vi "Create trap overlay.vi"(0 "Current trap cluster":T1, 1 "Image in":T2, 2 "ROI size":dbl=24.0, 3 "Switch X/Y":bool, 4 "Path":T1[](array[typedef])) -> (5 "Image Out":T2)   [LabVIEW 8.6]
uses:
  <vilib>/vision/Image Controls.llb/IMAQ Image.ctl
  Trap cluster.ctl
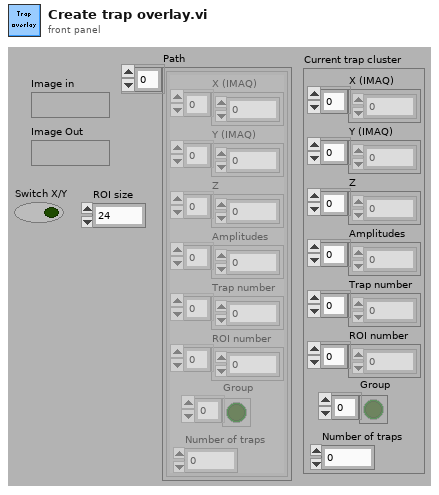
[diagram p1: front panel]
types:
  T1 = typedef "Trap cluster.ctl" = cluster{"X (IMAQ)":dbl[], "Y (IMAQ)":dbl[], "Z":dbl[], "Amplitudes":dbl[], "Trap number":i32[], "ROI number":i32[], "Number of traps":i32, "Group":bool[]}
  T2 = typedef "IMAQ Image.ctl" = refnum<image>
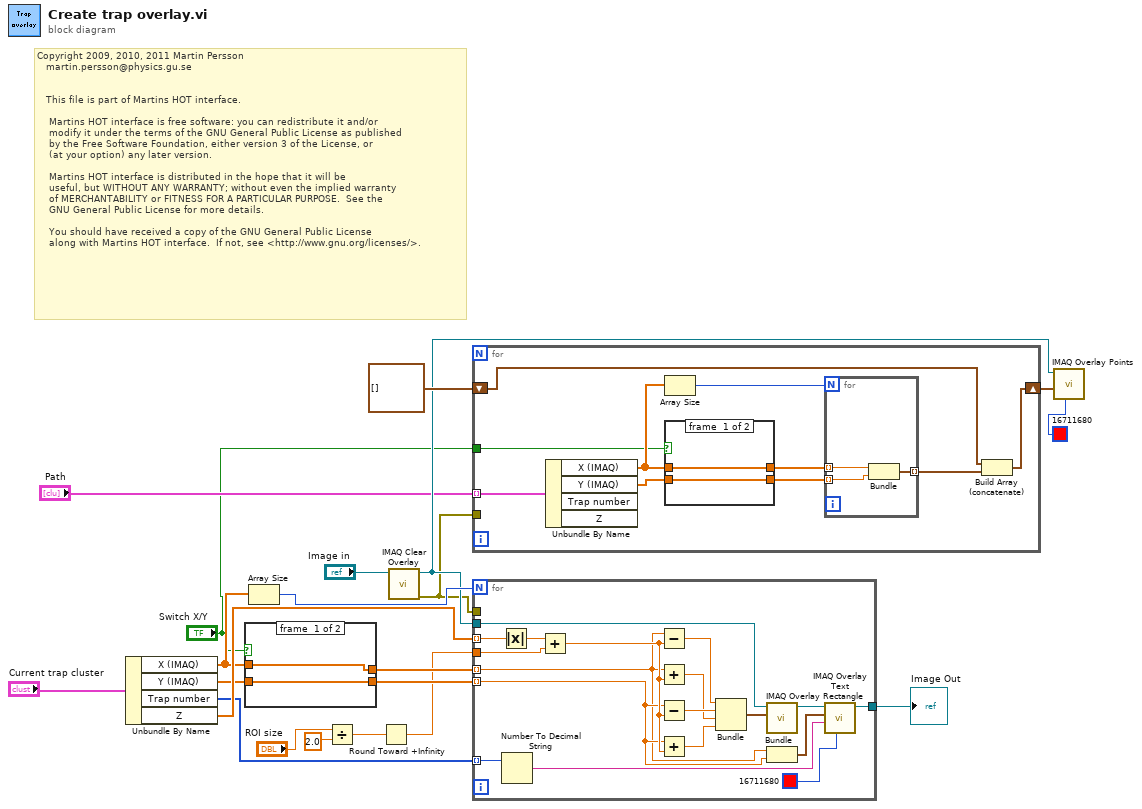
[diagram p0: block diagram]
diagram:
  # "Copyright 2009, 2010, 2011 Martin Persson \n   martin.persson@physics.gu.se\n\n\n   This file is part of Martins HOT interface.\n\n    Martins HOT interface is free software: you can redistribute it and/or \n    modify it under the terms of the GNU General Public License as published \n    by the Free Software Foundation, either version 3 of the License, or\n    (at your option) any later version.\n\n    Martins HOT interface is distributed in the hope that it will be \n    useful, but WITHOUT ANY WARRANTY; without even the implied warranty\n    of MERCHANTABILITY or FITNESS FOR A PARTICULAR PURPOSE.  See the\n    GNU General Public License for more details.\n\n    You should have received a copy of the GNU General Public License\n    along with Martins HOT interface.  If not, see <http://www.gnu.org/licenses/>."
  n1 = Unbundle By Name("Current trap cluster") -> ("X (IMAQ)"=w13:dbl[], "Y (IMAQ)"=w17:dbl[], "Trap number"=w20:i32[], "Z"=w21:dbl[])
  n2 = case shown="False" "Switch X/Y" {
    tunnel: w13 -> [w23 w25]
    tunnel: [w23 w24] -> w16
    tunnel: w17 -> [w22 w24]
    tunnel: [w22 w25] -> w15
    frame #0 {
    }
    frame #1 {
    }
  }
  n3 = Array Size(array=w13) -> (size(s)=w14:i32)
  n4 = Divide(x="ROI size", y=2.0) -> (x/y=w10:dbl)
  n5 = Round Toward +Infinity(x=w10) -> (ceil(x): smallest int >= x=w9:dbl)
  n6 = call "IMAQ Clear Overlay"("Image"="Image in") -> ("error out"=w3:errorcluster, "Image Out"=w6:T2)  [unwired: 9 in]
  n7 = for {
    tunnel: "Path" -> [w30] mode=indexing
    shift-right: [w28] -> w7
    shift-left: cluster{dbl, dbl}[] [] -> [w27]
    tunnel: w3 -> [_]
    tunnel: "Switch X/Y" -> [w26]
    n8 = Unbundle By Name(w30) -> ("X (IMAQ)"=w35:dbl[], "Y (IMAQ)"=w31:dbl[])  [unwired: 2 out]
    n9 = Array Size(array=w35) -> (size(s)=w34:i32)
    n10 = case shown="True" w26 {
      tunnel: w35 -> [w37 w39]
      tunnel: [w37 w38] -> w32
      tunnel: w31 -> [w36 w38]
      tunnel: [w36 w39] -> w33
      frame #0 {
      }
      frame #1 {
      }
    }
    n11 = for {
      N: w34 -> [_]
      tunnel: w32 -> [w41] mode=indexing
      tunnel: w33 -> [w42] mode=indexing
      tunnel: [w40] -> w29 mode=indexing
      n12 = Bundle(w41, w42) -> (w40:cluster{dbl, dbl})  [unwired: 1 in]
    }
    n13 = Build Array (concatenate)(w27, w29) -> (w28:cluster{dbl, dbl}[])
  }
  n14 = for {
    N: w14 -> [_]
    tunnel: w6 -> [w60]
    tunnel: w16 -> [w44] mode=indexing
    tunnel: w15 -> [w45] mode=indexing
    tunnel: w20 -> [w48] mode=indexing
    tunnel: w21 -> [w52] mode=indexing
    tunnel: [w50] -> w19
    tunnel: w9 -> [w43]
    tunnel: w3 -> [_]
    n15 = Absolute Value(x=w52) -> (abs(x)=w59:dbl)
    n16 = Number To Decimal String(number=w48) -> (decimal integer string=w47:string)  [unwired: 1 in]
    n17 = Add(x=w59, y=w43) -> (x+y=w58:dbl)
    n18 = Subtract(x=w44, y=w58) -> (x-y=w57:dbl)
    n19 = Add(x=w44, y=w58) -> (x+y=w55:dbl)
    n20 = Subtract(x=w45, y=w58) -> (x-y=w56:dbl)
    n21 = Add(x=w45, y=w58) -> (x+y=w54:dbl)
    n22 = Bundle(w57, w56, w55, w54) -> (w53:cluster{dbl, dbl, dbl, dbl})  [unwired: 1 in]
    n23 = call "IMAQ Overlay Rectangle"("Rectangle"=w53, "Image"=w60) -> ("Image Out"=w51:T2)  [unwired: 8 in, 1 out]
    n24 = Bundle(w44, w45) -> (w49:cluster{dbl, dbl})  [unwired: 1 in]
    n25 = call "IMAQ Overlay Text"("Text Color (black)"=u32 16711680, "String"=w47, "Origin"=w49, "Image"=w51) -> ("Image Out"=w50:T2)  [unwired: 6 in, 1 out]
  }
  "Image Out" <- w19
  n26 = call "IMAQ Overlay Points"("Color"=u32 16711680 ("Text Color (black)"), "Array of Points"=w7, "Image"=w6) -> ()  [unwired: 7 in, 2 out]
